vi "TextControlledInstrumMakeControlMap.vi"(8 "ValueMap in (empty)":map{string, variant}(c390), 9 "ControlMap in (empty)":map{string, refnum<vi>}(c390), 10 "Prefix (\"\")":string, 11 "ControlArray":refnum<vi>[](array[refnum])) -> (0 "ValueMap out":map{string, variant}(c390), 1 "ControlMap out":map{string, refnum<vi>}(c390), 2 "Names":string[](array[string]), 3 "Controls":refnum<vi>[](array[refnum]))   [LabVIEW 2021]
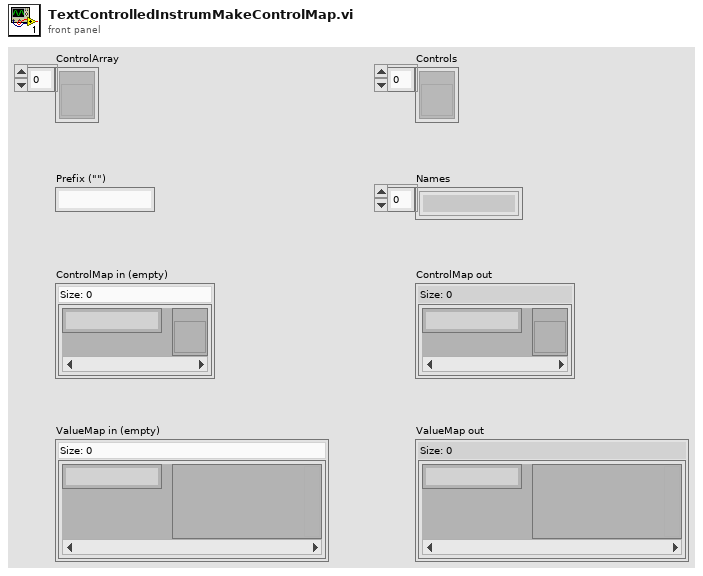
[diagram p1: front panel]
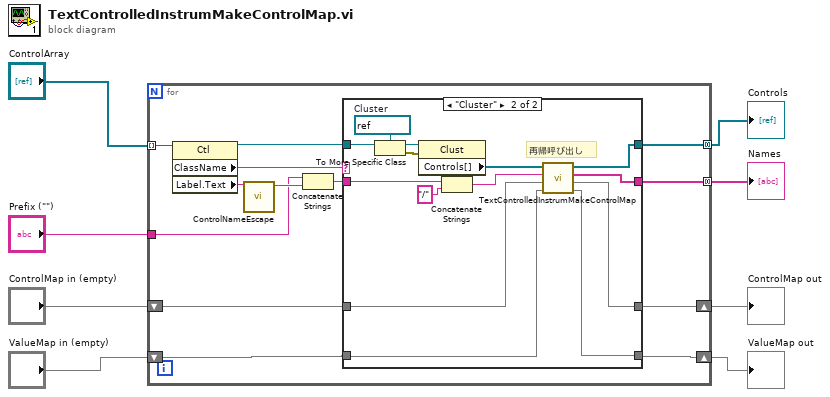
[diagram p0: block diagram]
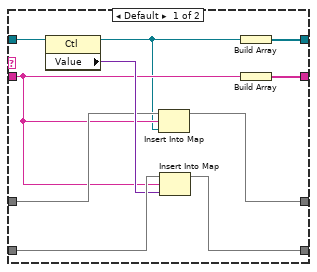
[diagram p2: hidden frame]
diagram:
  n1 = for {
    tunnel: "ControlArray" -> [w21] mode=indexing
    tunnel: "Prefix (\"\")" -> [w14]
    shift-right: [w12] -> w4
    shift-left: "ControlMap in (empty)" -> [w16]
    shift-right: [w11] -> w3
    shift-left: "ValueMap in (empty)" -> [w13]
    tunnel: [w10] -> w2 mode=concatenating
    tunnel: [w9] -> w1 mode=concatenating
    n2 = property class="Ctl"(reference=w21) -> (reference out=w19:refnum<vi>, "ClassName"=w20:string, "Label.Text"=w18:string)  [unwired: 1 in, 1 out]
    n3 = call "ControlNameEscape.vi"("label"=w18) -> ("escaped string"=w17:string)  [unwired: 10 in]
    n4 = Concatenate Strings(w14, w17) -> (w15:string)
    n5 = case shown="\"Cluster\"" w20 {
      tunnel: w19 -> [w31 w45]
      tunnel: w15 -> [w25 w38]
      tunnel: w16 -> [w27 w37]
      tunnel: w13 -> [w30 w36]
      tunnel: [w26 w35] -> w12
      tunnel: [w29 w34] -> w11
      tunnel: [w24 w33] -> w10
      tunnel: [w22 w32] -> w9
      frame Default {
        n6 = property class="Ctl"(reference=w31) -> (reference out=w23:refnum<vi>, "Value"=w28:variant)  [unwired: 1 in, 1 out]
        n7 = Insert Into Map(map in=w27, key=w25, value=w23) -> (map out=w26:map{string, refnum<vi>})  [unwired: 2 out]
        n8 = Insert Into Map(map in=w30, key=w25, value=w28) -> (map out=w29:map{string, variant})  [unwired: 2 out]
        n9 = Build Array(w23) -> (w22:refnum<vi>[])
        n10 = Build Array(w25) -> (w24:string[])
      }
      frame "Cluster" {
        w44 = refnum<vi> refnum  # Cluster
        # "再帰呼び出し"
        n11 = To More Specific Class(target class=w44, reference=w45) -> (specific class reference=w43:refnum<vi>, error out=w42:errorcluster)  [unwired: 1 in]
        n12 = property class="Clust"(reference=w43, error in=w42) -> ("Controls[]"=w41:refnum<vi>[])  [unwired: 2 out]
        n13 = Concatenate Strings(w38, "/" ("string")) -> (w40:string)
        n14 = call "TextControlledInstrumMakeControlMap.vi"("ValueMap in (empty)"=w36, "ControlMap in (empty)"=w37, "Prefix (\"\")"=w40, "ControlArray"=w41) -> ("ValueMap out"=w34:map{string, variant}, "ControlMap out"=w35:map{string, refnum<vi>}, "Names"=w33:string[], "Controls"=w32:refnum<vi>[])  [unwired: 4 in]
      }
    }
  }
  "ControlMap out" <- w4
  "ValueMap out" <- w3
  "Names" <- w2
  "Controls" <- w1
